vi "Close.vi"(8 "error in":errorcluster, 11 "4-20mA Settings In":T1) -> (0 "error out":errorcluster, 3 "4-20mA Settings Out":T1)   [LabVIEW 2021, in "Pressure Transmitter Library.lvlib"]
uses:
  Pressure Transmitter Library.lvlib
  Pressure Transmitter Device Settings.ctl
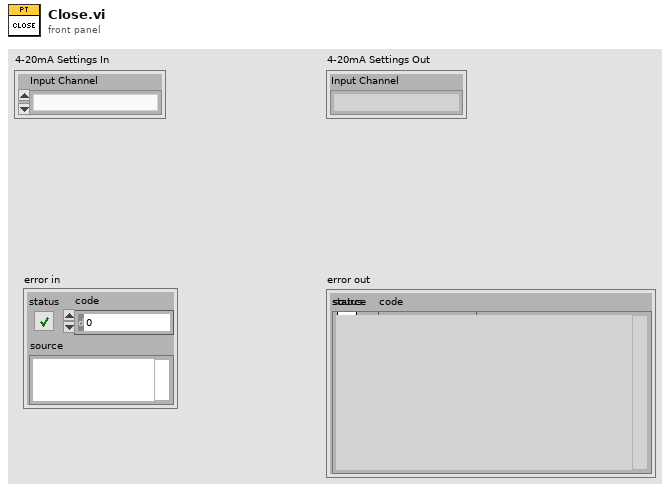
[diagram p1: front panel]
types:
  T1 = typedef "Pressure Transmitter Library.lvlib/Pressure Transmitter Device Settings.ctl" = cluster{"Input Channel ":u16}
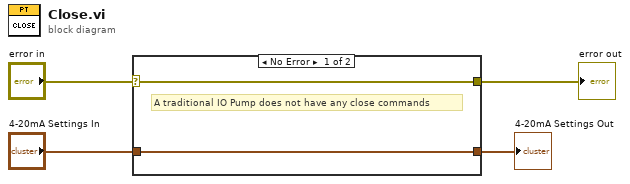
[diagram p0: block diagram]
diagram:
  n1 = case shown="No Error" "error in" {
    selector: "error in" -> [w6 w8]
    tunnel: [w6 w8] -> w3
    tunnel: "4-20mA Settings In" -> [w5 w7]
    tunnel: [w5 w7] -> w2
    frame No Error {
      # "A traditional IO Pump does not have any close commands"
    }
    frame Error {
    }
  }
  "error out" <- w3
  "4-20mA Settings Out" <- w2
